vi "Parse Thing Shadow JSON.vi"(11 "JSON":string) -> (1 "Version":i32, 2 "Reported State":T1[](array[typedef]), 3 "Desired State":T1[](array[typedef]))   [LabVIEW 2015, in "NI_AWS_IoT.lvlib"]
uses:
  NI_AWS_IoT.lvlib
  JSON Parsing/Name-Value with Type.ctl
  JSON Parsing/Name Value Pair.ctl
  JSON Parsing/JSON Type.ctl
  JSON Parsing/NI_JSON Parsing.lvlib
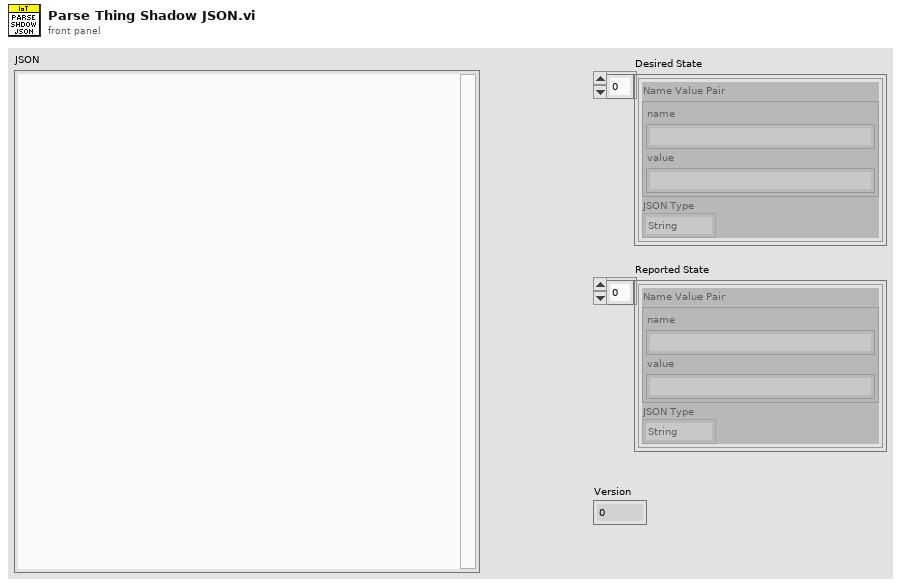
[diagram p1: front panel]
types:
  T1 = typedef "NI_JSON Parsing.lvlib/Name-Value with Type.ctl" = cluster{"Name Value Pair":T2, "JSON Type":T3}
  T2 = typedef "NI_JSON Parsing.lvlib/Name Value Pair.ctl" = cluster{"name":string, "value":string}
  T3 = typedef "NI_JSON Parsing.lvlib/JSON Type.ctl" = enum16{"String", "Numeric", "Boolean"}
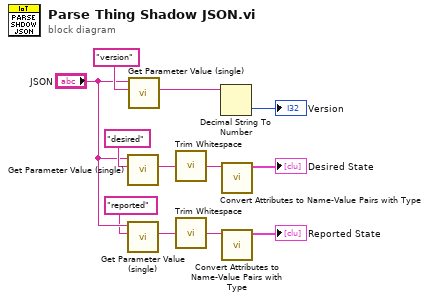
[diagram p0: block diagram]
diagram:
  n1 = call "Get Parameter Value (single).vi"("Parameter Name"="desired", "JSON"="JSON") -> ("Parameter Value"=w8:string)  [unwired: 6 in, 3 out]
  n2 = call "Get Parameter Value (single).vi"("Parameter Name"="reported", "JSON"="JSON") -> ("Parameter Value"=w4:string)  [unwired: 6 in, 3 out]
  n3 = call "Get Parameter Value (single).vi"("Parameter Name"="version", "JSON"="JSON") -> ("Parameter Value"=w11:string)  [unwired: 6 in, 3 out]
  n4 = call <vilib>:"Trim Whitespace.vi"("string"=w8) -> ("trimmed string"=w7:string)  [unwired: 1 in]
  n5 = call <vilib>:"Trim Whitespace.vi"("string"=w4) -> ("trimmed string"=w5:string)  [unwired: 1 in]
  n6 = Decimal String To Number(string=w11) -> (number=→"Version":i32)  [unwired: 2 in, 1 out]
  n7 = call "Convert Attributes to Name-Value Pairs with Type.vi"("JSON Attributes"=w7) -> ("Name-Value Pairs"=→"Desired State":T1[])  [unwired: 10 in]
  n8 = call "Convert Attributes to Name-Value Pairs with Type.vi"("JSON Attributes"=w5) -> ("Name-Value Pairs"=→"Reported State":T1[])  [unwired: 10 in]
